vi "NavXInfo.vi"(0 "error in":errorcluster) -> (1 "Board Information":T3 {"Board"."Hardware Revision" items=["navX-MXP"=33, "navX-Micro"=40]; "Omnimount Config" items=["DEFAULT", "X_UP", "X_DOWN", "Y_UP", "Y_DOWN", "Z_UP", "Z_DOWN"]}, 2 "error out":errorcluster)   [LabVIEW 2017]
uses:
  <vilib>/Rock Robotics/WPI/ThirdParty/Sensors/navX/_TypeDefs/Flags/Z900_navX_Flags_HardwareRevTypeDef.ctl
  <vilib>/Rock Robotics/WPI/ThirdParty/Sensors/navX/_TypeDefs/Flags/Z900_navX_Flags_OmnimountConfigTypeDef.ctl
  <vilib>/Rock Robotics/Network Tables/NT Write Numeric Array.vi
  <vilib>/Rock Robotics/Network Tables/NT Write Number.vi
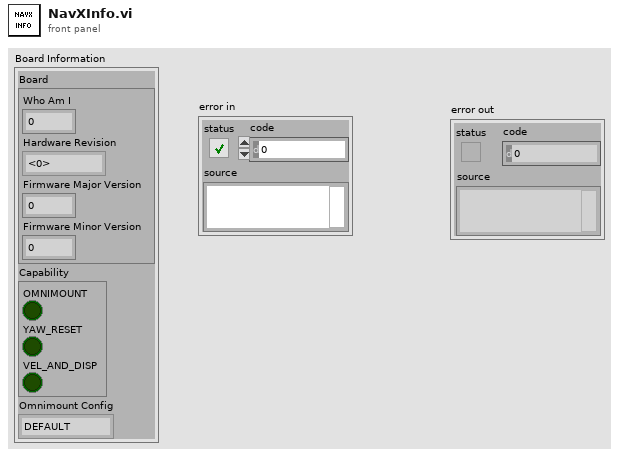
[diagram p1: front panel]
types:
  T1 = typedef "Z900_navX_Flags_HardwareRevTypeDef.ctl" = u8
  T2 = typedef "Z900_navX_Flags_OmnimountConfigTypeDef.ctl" = u8
  T3 = cluster{"Board":cluster{"Who Am I":u8, "Hardware Revision":T1, "Firmware Major Version":u8, "Firmware Minor Version":u8}, "Capability":cluster{"OMNIMOUNT":bool, "YAW_RESET":bool, "VEL_AND_DISP":bool}, "Omnimount Config":T2}
  T4 = cluster{"Yaw":dbl, "Roll":dbl, "Pitch":dbl, "Heading":dbl, "Fused Heading":dbl}
  T5 = cluster{"LinearAcceleration X":dbl, "LinearAcceleration Y":dbl, "LinearAcceleration Z":dbl}
  T6 = cluster{"Velocity X":dbl, "Velocity Y":dbl, "Velocity Z":dbl, "Displacement X":dbl, "Displacement Y":dbl, "Displacement Z":dbl}
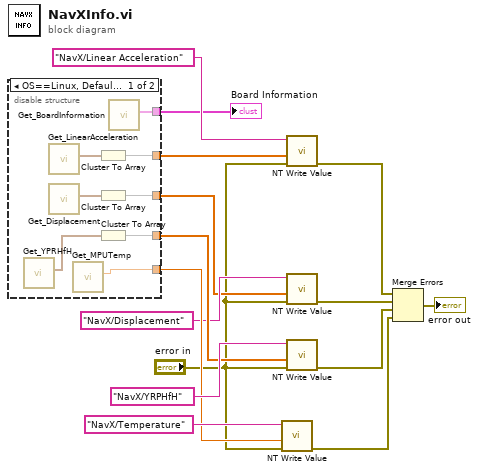
[diagram p0: block diagram]
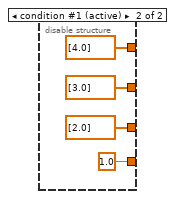
[diagram p2: hidden frame]
diagram:
  n1 = disable-structure shown="OS==Linux, Default" {
    disable-tunnel: [w23 dbl[] [2.0] ("YRPHfH")] -> w14
    disable-tunnel: [w16 1.0 ("MPUTemp")] -> w12
    disable-tunnel: [w22 dbl[] [4.0] ("Linear Acceleration")] -> w10
    disable-tunnel: [w20 dbl[] [3.0] ("Displacement")] -> w8
    disable-tunnel: [w18 _] -> w7
    frame condition #0 {
      n2 = call <vilib>:"Get_YPRHfH.vi"() -> ("YRPHfH"=w17:T4)  [unwired: 11 in]
      n3 = call <vilib>:"Get_LinearAcceleration.vi"() -> ("Linear Acceleration"=w21:T5)  [unwired: 11 in]
      n4 = call <vilib>:"Get_Displacement.vi"() -> ("Displacement"=w19:T6)  [unwired: 11 in]
      n5 = call <vilib>:"Get_MPUTemp.vi"() -> ("MPUTemp"=w16:dbl)  [unwired: 11 in]
      n6 = Cluster To Array(cluster=w21) -> (array=w22:dbl[])
      n7 = Cluster To Array(cluster=w19) -> (array=w20:dbl[])
      n8 = Cluster To Array(cluster=w17) -> (array=w23:dbl[])
      n9 = call <vilib>:"Get_BoardInformation.vi"() -> ("Board Information"=w18:T3)  [unwired: 11 in]
    }
    frame condition #1 (active) {
    }
  }
  "Board Information" <- w7
  n10 = call-poly <vilib>:"NT Write Value.vi"("error in"="error in", "Numeric"=w12, "Name"="NavX/Temperature") -> ("error out"=w2:errorcluster)  [unwired: 8 in]
  n11 = call-poly <vilib>:"NT Write Value.vi"("error in"="error in", "Numeric Array"=w10, "Name"="NavX/Linear Acceleration") -> ("error out"=w5:errorcluster)  [unwired: 8 in]
  n12 = call-poly <vilib>:"NT Write Value.vi"("error in"="error in", "Numeric Array"=w8, "Name"="NavX/Displacement") -> ("error out"=w4:errorcluster)  [unwired: 8 in]
  n13 = call-poly <vilib>:"NT Write Value.vi"("error in"="error in", "Numeric Array"=w14, "Name"="NavX/YRPHfH") -> ("error out"=w3:errorcluster)  [unwired: 8 in]
  n14 = Merge Errors(w5, w4, w3, w2) -> (→"error out":errorcluster)
